vi "Create Event Type-Def.vi"() -> ()   [LabVIEW 2018, in "Scripting.lvlib"]
uses:
  Scripting/Locale-Strings.ctl
  <vilib>/Utility/traverseref.llb/TRef TravTarget.ctl
  Scripting.lvlib
  <vilib>/Utility/traverseref.llb/VI Scripting - Traverse.lvlib
panel:
  in  "error in (no error)":errorcluster
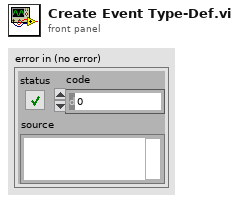
[diagram p1: front panel]
types:
  T1 = enum32{"Invalid", "Standard", "Closed", "Hidden", "Minimized", "Maximized"}
  T2 = typedef "TRef TravTarget.ctl" = enum16{"FP", "BD", "Other"}
  T3 = typedef "Scripting.lvlib/Locale-Strings.ctl" = enum16{"Event-Type-Def-Creation-API-Call"}
  T4 = enum32{"invalid VI type", "Standard VI", "Control VI", "Global VI", "Polymorphic VI", "Configuration VI", "SubSystem", "Facade VI", "Method VI", "Statechart Diagram VI"}
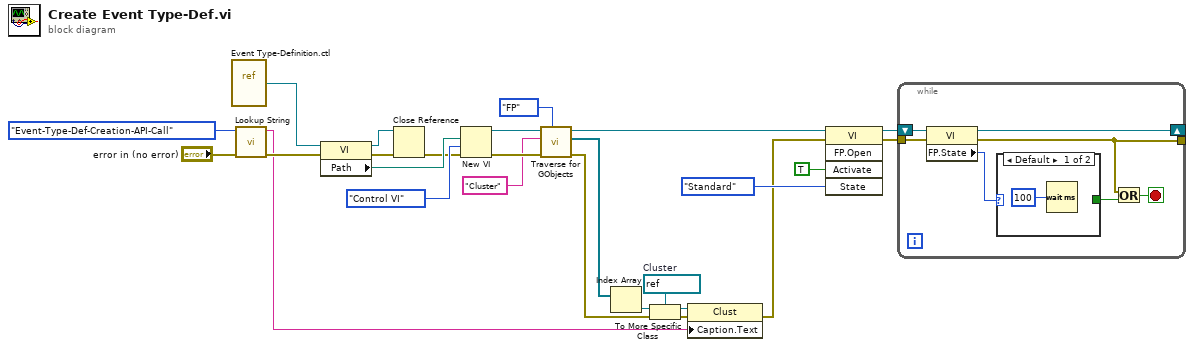
[diagram p0: block diagram]
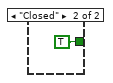
[diagram p2: hidden frame]
diagram:
  w11 = refnum<vi> refnum  # Cluster
  n1 = vi-ref "Event Type-Definition.ctl"() -> (w25:refnum<vi>)
  n2 = call "Lookup String.vi"("error in (no error)"="error in (no error)", "Locale String"=Locale-Strings."Event-Type-Def-Creation-API-Call") -> ("error out"=w19:errorcluster, "String"=w7:string)  [unwired: 8 in]
  n3 = property class="VI"(reference=w25, error in=w19) -> (reference out=w21:refnum<vi>, error out=w23:errorcluster, "Path"=w24:path)
  n4 = Close Reference(reference=w21, error in (no error)=w23) -> (error out=w22:errorcluster)
  n5 = New VI(8:w22, 9:T4."Control VI" ("vi type (standard vi)"), 10:w24) -> (0:w17:errorcluster, 3:w16:refnum<vi>)  [unwired: 4 in]
  n6 = call <vilib>:"Traverse for GObjects.vi"("Traverse Target"=TRef_TravTarget."FP", "error in (no error)"=w17, "Class Name"="Cluster", "VI Refnum"=w16) -> ("error out"=w10:errorcluster, "References"=w13:refnum<vi>[], "dup VI Refnum"=w4:refnum<vi>)  [unwired: 4 in, 1 out]
  n7 = Index Array(array=w13) -> (element=w12:refnum<vi>)  [unwired: 1 in]
  n8 = To More Specific Class(target class=w11, reference=w12, error in=w10) -> (specific class reference=w8:refnum<vi>, error out=w9:errorcluster)
  n9 = property class="Clust"(reference=w8, error in=w9, "Caption.Text"=w7) -> (error out=w3:errorcluster)  [unwired: 1 out]
  n10 = invoke class="VI" method="FP.Open"(reference=w4, error in=w3, "Activate"=TRUE ("Activate?"), "State"=T1."Standard") -> (reference out=w2:refnum<vi>, error out=w1:errorcluster)  [unwired: 1 in, 3 out]
  n11 = while {
    tunnel: w1 -> [w32]
    shift-right: [w29] -> _
    shift-left: w2 -> [w33]
    tunnel: [w27] -> _
    stop <- w28 stop-if-true
    n12 = property class="VI"(reference=w33, error in=w32) -> (reference out=w29:refnum<vi>, error out=w27:errorcluster, "FP.State"=w31:T1)
    n13 = case shown="Default" w31 {
      tunnel: [_ TRUE] -> w30
      frame Default {
        n14 = Wait (ms)(milliseconds to wait=u32 100) -> ()  [unwired: 1 out]
      }
      frame "Closed" {
      }
    }
    n15 = Or(x=w27, y=w30) -> (x .or. y?=w28:bool)
  }
